vi "CRYPlot Polar Graph.vi"(7 "pGraph VI In":refnum<vi>, 8 "sOption":string, 9 "GraphSet":bool, 10 "Flattened Polar Property":string="Polar Property", 11 "Selected Rows In":i32[](array[numeric])) -> (0 "ItemSyms":i32[](array[numeric]), 1 "Freq Color":u32[](array[numeric]), 2 "Freq Name":string[](array[string]), 3 "Selected Row Out":i32[](array[numeric]))   [LabVIEW 2013]
uses:
  CRYWindow/DataView/Control/CRYPolar Property.ctl
  Global/CRYCurve Library Global.vi
panel:
  in  "Polar Property":T1={"polar attributes"={"maximum"=2.0, "minimum"=0.0, "clip to min"=FALSE, "log"=FALSE, "grid color"=3381657, "plot color"=16711680, "fmt and prec"={"format"=enum."Decimal", "precision"=2}, "visible section"=4}, "Auto/Manual"=0, "Zero Adjust (deg)"=0, "Angle Increment (deg)"=0, "Mirror"=FALSE, "Auto Increment"=FALSE, "Total Rotatin (deg)"=0, "Discrete/Rannge"=0, "Show Name"=FALSE, "CurValues"=[], "CurIndex"=0, "CurColors"=[], "CurColors_Range"=[], "CurValues_Range"=[], "Pen"={"Width"=1, "Style"=enum."Solid"}, "BackgroundColor"=0} {"polar attributes"."minimum" format="%0.2f"; "polar attributes"."maximum" format="%0.2f"}
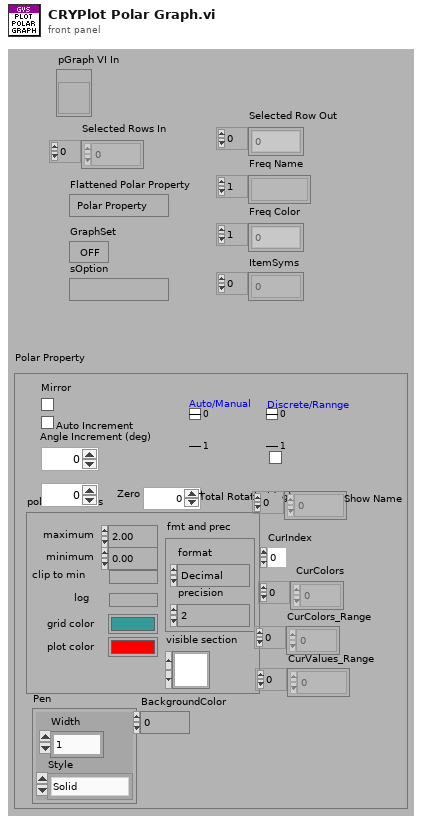
[diagram p1: front panel]
types:
  T1 = typedef "CRYPolar Property.ctl" = cluster{"polar attributes":cluster{"maximum":dbl, "minimum":dbl, "clip to min":bool, "log":bool, "grid color":u32, "plot color":u32, "fmt and prec":cluster{"format":enum8{"Decimal", "Scientific", "Engineering", "Binary", "Octal", "Hex"}, "precision":u8}, "visible section":u16}, "Auto/Manual":u16, "Zero Adjust (deg)":i32, "Angle Increment (deg)":i32, "Mirror":bool, "Auto Increment":bool, "Total Rotatin (deg)":i32, "Discrete/Rannge":u16, "Show Name":bool, "CurValues":dbl[], "CurIndex":u16, "CurColors":u32[], "CurColors_Range":u32[], "CurValues_Range":dbl[], "Pen":cluster{"Width":u16, "Style":enum32{"Solid", "Dash", "Dot", "DashDot", "DashDotDot"}}, "BackgroundColor":u32}
  T2 = cluster{"left":i16, "top":i16, "right":i16, "bottom":i16}
  T3 = typedef "CRYData Cluster.ctl" = cluster{"Name":string, "Curve":cluster{"x":dbl, "y":dbl, "z":dbl}[], "X data":u16, "Y data":u16, "Z data":u16, "X axis":u16, "Y axis":u16, "Z axis":u16, "X unit":string, "Y unit":string, "Z unit":string, "X dB ref":dbl, "Y dB ref":dbl, "Z dB ref":dbl, "single val":bool, "protected":bool, "display X":bool, "display Y":bool, "display Z":bool, "Test Info":string, "Step No.":i32, "Plot Settings":cluster{"Color":u32, "Interpolation":u8, "Point Style":u8, "Line Style":u8, "Point Color":u32, "Line Width":u8, "Bar Plot Style":u8, "Fill To":i16}, "AutoProtect":bool}
  T4 = cluster{"maximum":dbl, "minimum":dbl, "clip to min":bool, "log":bool, "grid color":u32, "plot color":u32, "fmt and prec":cluster{"format":enum8{"Decimal", "Scientific", "Engineering", "Binary", "Octal", "Hex"}, "precision":u8}, "visible section":u16}
  T5 = cluster{"Width":u16, "Style":enum32{"Solid", "Dash", "Dot", "DashDot", "DashDotDot"}}
  T6 = typedef "LVBoundsTypeDef.ctl" = cluster{"Width":u32, "Height":u32}
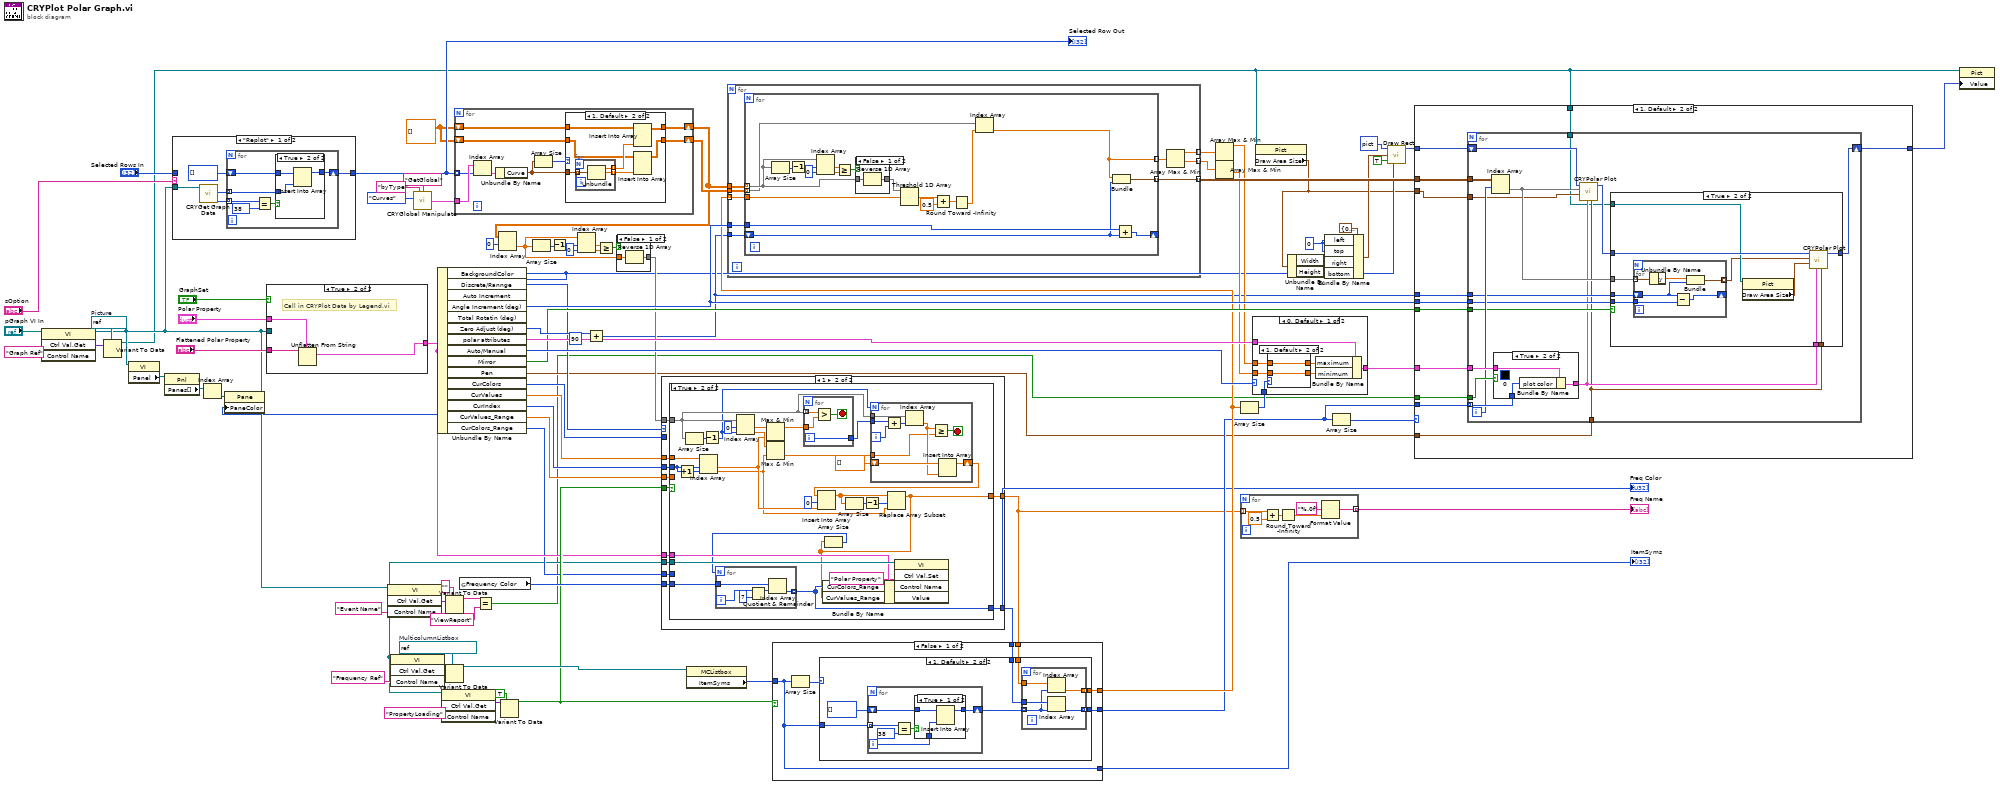
[diagram p0: block diagram]
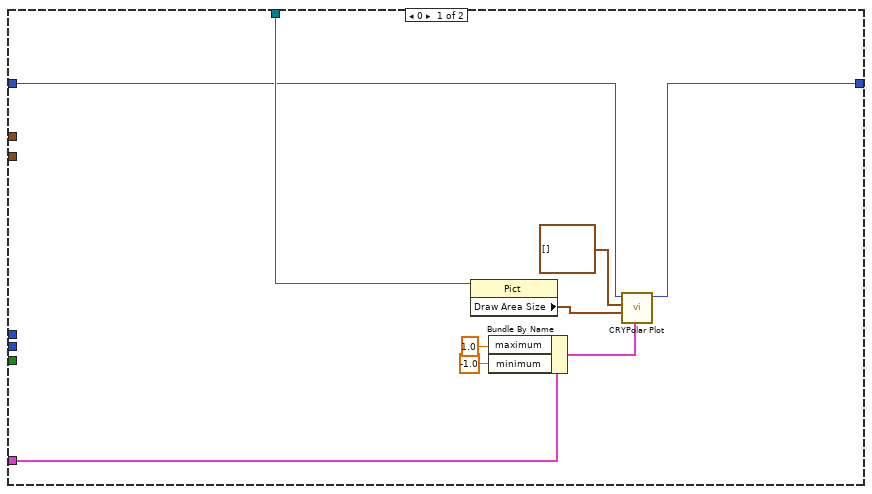
[diagram p6: hidden frame]
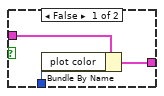
[diagram p8: hidden frame]
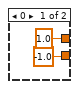
[diagram p11: hidden frame]
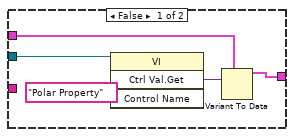
[diagram p17: hidden frame]
diagram:
  w13 = i16 0 ("left")
  w25 = refnum<vi> refnum  # Picture
  w32 = dbl[][] []
  w70 = refnum<vi> refnum  # MulticolumnListbox
  n1 = invoke class="VI" method="Ctrl Val.Get"(reference="pGraph VI In", "Control Name"="Graph Ref") -> (reference out=w21:refnum<vi>, "Get Control Value Variant"=w24:variant)  [unwired: 2 in, 2 out]
  n2 = Variant To Data(type=w25, Variant=w24) -> (data=w9:refnum<vi>)  [unwired: 1 in, 1 out]
  n3 = property class="VI"(reference=w21) -> ("Panel"=w19:refnum<vi>)  [unwired: 1 in, 2 out]
  n4 = property class="Pnl"(reference=w19) -> ("Panes[]"=w18:refnum<vi>[])  [unwired: 1 in, 2 out]
  n5 = case shown="\"Replot\"" "sOption" {
    tunnel: w21 -> [w89 _]
    tunnel: [w88 w103] -> w67
    tunnel: "Selected Rows In" -> [_ w103]
    frame "Replot" {
      n6 = call "CRYGet Graph Data.vi"("pGraph VI"=w89) -> ("Item Symbols"=w91:i32[], "Rows"=w92:i32[])  [unwired: 2 in, 7 out]
      n7 = for {
        tunnel: w91 -> [w97] mode=indexing
        tunnel: w92 -> [w95] mode=indexing
        shift-right: [w93] -> w88
        shift-left: i32[] [] ("Rows") -> [w94]
        n8 = Equal?(x=w97, y=38) -> (x = y?=w96:bool)
        n9 = case shown="True" w96 {
          tunnel: w95 -> [_ w100]
          tunnel: w94 -> [w99 w102]
          tunnel: [w99 w101] -> w93
          frame False {
          }
          frame True {
            n10 = Insert Into Array(array=w102, new element=w100) -> (w101:i32[])  [unwired: 1 in]
          }
        }
      }
    }
    frame "SameDrop", Default {
    }
  }
  "Selected Row Out" <- w67
  n11 = Index Array(array=w18) -> (element=w17:refnum<vi>)  [unwired: 1 in]
  n12 = case shown="True" "GraphSet" {
    tunnel: [w108 w109] -> w59
    tunnel: "Polar Property" -> [w107 w110]
    tunnel: w21 -> [w106 _]
    tunnel: "Flattened Polar Property" -> [_ w111]
    frame False {
      n13 = invoke class="VI" method="Ctrl Val.Get"(reference=w106, "Control Name"="Polar Property") -> ("Get Control Value Variant"=w104:variant)  [unwired: 2 in, 3 out]
      n14 = Variant To Data(type=w107, Variant=w104) -> (data=w108:T1)  [unwired: 1 in, 1 out]
    }
    frame True {
      # "Call in CRYPlot Data by Legend.vi"
      n15 = Unflatten From String(type=w110, binary string=w111) -> (value=w109:T1)  [unwired: 3 in, 2 out]
    }
  }
  n16 = invoke class="VI" method="Ctrl Val.Get"(reference=w21, "Control Name"="Event Name") -> ("Get Control Value Variant"=w83:variant)  [unwired: 2 in, 3 out]
  n17 = invoke class="VI" method="Ctrl Val.Get"(reference=w21, "Control Name"="Frequency Ref") -> ("Get Control Value Variant"=w71:variant)  [unwired: 2 in, 3 out]
  n18 = call "CRYGlobal Manipulate.vi"("Type"=enum16{"Curves", "Values", "Results", "WFM"}."Curves", "sOption"="byType", "sAction"="GetGlobal") -> ("Curves Out"=w1:T3[])  [unwired: 6 in, 6 out]
  n19 = Unbundle By Name(w59) -> ("BackgroundColor"=w7:u32, "Discrete/Rannge"=w73:u16, "Angle Increment (deg)"=w79:i32, "Zero Adjust (deg)"=w78:i32, "polar attributes"=w77:T4, "Auto/Manual"=w76:u16, "Mirror"=w75:bool, "Pen"=w28:T5, "CurColors"=w29:u32[], "CurValues"=w74:dbl[], "CurIndex"=w61:u16, "CurValues_Range"=w60:dbl[], "CurColors_Range"=w58:u32[])  [unwired: 2 out]
  n20 = property class="Pane"(reference=w17, "PaneColor"=w7) -> ()  [unwired: 1 in, 2 out]
  n21 = invoke class="VI" method="Ctrl Val.Get"(reference=w21, "Control Name"="PropertyLoading") -> ("Get Control Value Variant"=w64:variant)  [unwired: 2 in, 3 out]
  n22 = Variant To Data(type=w70, Variant=w71) -> (data=w69:refnum<vi>)  [unwired: 1 in, 1 out]
  n23 = Variant To Data(type="" ("Control Name"), Variant=w83) -> (data=w81:string)  [unwired: 1 in, 1 out]
  n24 = for {
    tunnel: w1 -> [w120]
    tunnel: w67 -> [w119] mode=indexing
    shift-right: [w113] -> w30
    shift-left: w32 -> [w115]
    shift-right: [w112] -> w31
    shift-left: w32 -> [w114]
    n25 = Index Array(array=w120, index=w119) -> (element=w118:T3)
    n26 = Unbundle By Name(w118) -> ("Curve"=w117:cluster{"x":dbl, "y":dbl, "z":dbl}[])
    n27 = Array Size(array=w117) -> (size(s)=w116:i32)
    n28 = case shown="1, Default" w116 {
      tunnel: w117 -> [_ w129]
      tunnel: w115 -> [w122 w128]
      tunnel: w114 -> [w121 w126]
      tunnel: [w122 w124] -> w113
      tunnel: [w121 w123] -> w112
      frame 0 {
      }
      frame 1, Default {
        n29 = for {
          tunnel: w129 -> [w132] mode=indexing
          tunnel: [w131] -> w125 mode=indexing
          tunnel: [w130] -> w127 mode=indexing
          n30 = Unbundle(w132) -> ("x"=w130:dbl, "y"=w131:dbl)  [unwired: 1 out]
        }
        n31 = Insert Into Array(array=w128, new element=w127) -> (w124:dbl[][])  [unwired: 2 in]
        n32 = Insert Into Array(array=w126, new element=w125) -> (w123:dbl[][])  [unwired: 2 in]
      }
    }
  }
  n33 = global read "CRYCurve Library Global.vi" "Frequency Color"() -> (w68:u32[])
  n34 = Equal?(x=w81, y="ViewReport" ("regular expression")) -> (x = y?=w20:bool)
  n35 = Index Array(array=w30, index (row)=0) -> (element=w34:dbl[])  [unwired: 1 in]
  n36 = Variant To Data(type=TRUE, Variant=w64) -> (data=w62:bool)  [unwired: 1 in, 1 out]
  n37 = Array Size(array=w34) -> (size(s)=w35:i32)
  n38 = Decrement(x=w35) -> (x-1=w36:i32)
  n39 = Index Array(array=w34, index #1=w36, index #2=0 ("index")) -> (element #1=w39:dbl, element #2=w38:dbl)
  n40 = Add(x=w78, y=90) -> (x+y=w27:i32)
  n41 = Greater Or Equal?(x=w39, y=w38) -> (x >= y?=w40:bool)
  n42 = case shown="False" w40 {
    tunnel: w34 -> [w134 w135]
    tunnel: [w133 w135] -> w33
    frame False {
      n43 = Reverse 1D Array(array=w134) -> (reversed array=w133:dbl[])
    }
    frame True {
    }
  }
  n44 = case shown="1" w73 {
    tunnel: w74 -> [w137 w147]
    tunnel: w29 -> [w136 _]
    tunnel: w68 -> [_ w146]
    tunnel: [w137 w142] -> w44
    tunnel: w61 -> [_ w148]
    tunnel: [w136 w145] -> w43
    tunnel: w62 -> [_ w139]
    tunnel: w58 -> [_ w140]
    tunnel: w21 -> [_ w144]
    tunnel: w59 -> [_ w143]
    tunnel: w60 -> [_ w141]
    tunnel: w33 -> [_ w138]
    frame 0, Default {
    }
    frame 1 {
      n45 = case shown="True" w139 {
        tunnel: w148 -> [_ w171]
        tunnel: w147 -> [_ w178]
        tunnel: w146 -> [_ w177]
        tunnel: [w149 w176] -> w145
        tunnel: w144 -> [_ w175]
        tunnel: w143 -> [_ w174]
        tunnel: [w150 w152] -> w142
        tunnel: w141 -> [w150 _]
        tunnel: w140 -> [w149 _]
        tunnel: w138 -> [_ w162]
        frame False {
        }
        frame True {
          n46 = Increment(x=w171) -> (x+1=w170:u16)
          n47 = Array Size(array=w162) -> (size(s)=w167:i32)
          n48 = Index Array(array=w178, index #1=w171, index #2=w170) -> (element #1=w156:dbl, element #2=w154:dbl)
          n49 = Decrement(x=w167) -> (x-1=w160:i32)
          n50 = Index Array(array=w162, index #1=0 ("index"), index #2=w160) -> (element #1=w168:dbl, element #2=w166:dbl)
          n51 = Max & Min(x=w168, y=w156) -> (max(x,y)=w163:dbl)  [unwired: 1 out]
          n52 = Max & Min(x=w166, y=w154) -> (min(x,y)=w164:dbl)  [unwired: 1 out]
          n53 = for {
            tunnel: w163 -> [w190]
            tunnel: w162 -> [w191] mode=indexing
            tunnel: [w188] -> w165
            i -> [w188]
            stop <- w189 stop-if-true
            n54 = Greater?(x=w191, y=w190) -> (0:w189:bool)
          }
          n55 = for {
            N: w160 -> [_]
            tunnel: w162 -> [w187]
            tunnel: w165 -> [w186]
            tunnel: w164 -> [w179]
            shift-right: [w182] -> w157
            shift-left: dbl[] [] -> [w183]
            i -> [w181]
            stop <- w184 stop-if-true
            n56 = Add(x=w186, y=w181) -> (x+y=w185:i32)
            n57 = Index Array(array=w187, index=w185) -> (element=w180:dbl)
            n58 = Greater Or Equal?(x=w180, y=w179) -> (x >= y?=w184:bool)
            n59 = Insert Into Array(array=w183, new element=w180) -> (w182:dbl[])  [unwired: 1 in]
          }
          n60 = Insert Into Array(array=w157, index=0, new element=w156) -> (w151:dbl[])
          n61 = Array Size(array=w151) -> (size(s)=w155:i32)
          n62 = Decrement(x=w155) -> (x-1=w153:i32)
          n63 = Replace Array Subset(array=w151, new element=w154, index=w153) -> (w152:dbl[])
          n64 = Array Size(array=w152) -> (size(s)=w161:i32)
          n65 = for {
            N: w161 -> [_]
            tunnel: w177 -> [w194]
            tunnel: [w193] -> w176 mode=indexing
            i -> [w192]
            n66 = Quotient & Remainder(x=w192, y=7) -> (x-y*floor(x/y)=w196:i32)  [unwired: 1 out]
            n67 = Index Array(array=w194, index=w196) -> (element=w193:u32)
          }
          n68 = Bundle By Name(cluster=w174, "CurColors_Range"=w176, "CurValues_Range"=w152) -> (w172:T1)
          n69 = invoke class="VI" method="Ctrl Val.Set"(reference=w175, "Control Name"="Polar Property", "Value"=w172) -> ()  [unwired: 2 in, 5 out]
        }
      }
    }
  }
  "Freq Color" <- w43
  n70 = property on="Property Node" class="MCListbox"(reference=w69) -> ("ItemSyms"=w42:i32[])  [unwired: 1 in, 2 out]
  n71 = case shown="False" w62 {
    tunnel: [w202 w229] -> w48
    tunnel: w44 -> [w200 w229]
    tunnel: [w199 w228] -> w46
    tunnel: w43 -> [w198 w228]
    tunnel: [w197 w227] -> w45
    tunnel: w42 -> [w197 w227]
    frame False {
      n72 = Array Size(array=w197) -> (size(s)=w201:i32)
      n73 = case shown="1, Default" w201 {
        tunnel: w200 -> [w204 w211]
        tunnel: [w204 w210] -> w202
        tunnel: w198 -> [w203 w209]
        tunnel: [w203 w208] -> w199
        tunnel: w197 -> [_ w205]
        frame 0 {
        }
        frame 1, Default {
          n74 = for {
            tunnel: w205 -> [w221] mode=indexing
            shift-right: [w218] -> w206
            shift-left: i32[] [] ("Rows") -> [w219]
            i -> [w217]
            n75 = Equal?(x=w221, y=38) -> (x = y?=w220:bool)
            n76 = case shown="True" w220 {
              tunnel: w219 -> [w225 w226]
              tunnel: [w224 w226] -> w218
              tunnel: w217 -> [w223 _]
              frame True {
                n77 = Insert Into Array(array=w225, new element=w223) -> (w224:i32[])  [unwired: 1 in]
              }
              frame False {
              }
            }
          }
          n78 = for {
            tunnel: w206 -> [w212] mode=indexing
            tunnel: w211 -> [w216]
            tunnel: [w215] -> w210 mode=indexing
            tunnel: w209 -> [w214]
            tunnel: [w213] -> w208 mode=indexing
            n79 = Index Array(array=w216, index=w212) -> (element=w215:dbl)
            n80 = Index Array(array=w214, index=w212) -> (element=w213:u32)
          }
        }
      }
    }
    frame True {
      # "Property dialog has been currently loaded"
    }
  }
  "ItemSyms" <- w45
  n81 = for {
    tunnel: w27 -> [w238]
    tunnel: w79 -> [w237]
    tunnel: w48 -> [w236] mode=indexing
    tunnel: w31 -> [w235]
    tunnel: [w234] -> w55 mode=indexing
    tunnel: [w232] -> w54 mode=indexing
    tunnel: [w231] -> w53 mode=indexing
    tunnel: w30 -> [w230]
    n82 = for {
      tunnel: w235 -> [w240] mode=indexing
      tunnel: w236 -> [w243]
      tunnel: w237 -> [w247]
      shift-right: [w246] -> _
      shift-left: w238 -> [w245]
      tunnel: [w244] -> w234 mode=indexing
      tunnel: [w239] -> w233 mode=indexing
      tunnel: w230 -> [w241] mode=indexing
      n83 = Array Size(array=w241) -> (size(s)=w257:i32)
      n84 = Decrement(x=w257) -> (x-1=w256:i32)
      n85 = Index Array(array=w241, index #1=w256, index #2=0 ("index")) -> (element #1=w253:dbl, element #2=w254:dbl)
      n86 = Greater Or Equal?(x=w253, y=w254) -> (x >= y?=w249:bool)
      n87 = case shown="False" w249 {
        tunnel: w241 -> [w259 w260]
        tunnel: [w258 w260] -> w242
        frame False {
          n88 = Reverse 1D Array(array=w259) -> (reversed array=w258:dbl[])
        }
        frame True {
        }
      }
      n89 = Threshold 1D Array(2:w243, 3:w242) -> (0:w252:dbl)  [unwired: 1 in]
      n90 = Add(x=w252, y=0.5) -> (x+y=w250:dbl)
      n91 = Round Toward -Infinity(1:w250) -> (0:w248:dbl)
      n92 = Index Array(array=w240, index=w248) -> (element=w239:dbl)
      n93 = Bundle("y"=w239, w245) -> (w244:cluster{"y":dbl, i32})  [unwired: 1 out]
      n94 = Add(x=w247, y=w245) -> (x+y=w246:i32)
    }
    n95 = Array Max & Min(array=w233) -> (max value=w232:dbl, min value=w231:dbl)  [unwired: 2 out]
  }
  n96 = Array Max & Min(array=w54) -> (max value=w51:dbl)  [unwired: 3 out]
  n97 = Array Max & Min(array=w53) -> (min value=w50:dbl)  [unwired: 3 out]
  n98 = Array Size(array=w48) -> (size(s)=w49:i32)
  n99 = for {
    tunnel: w44 -> [w261] mode=indexing
    tunnel: [w265] -> w56 mode=indexing
    n100 = Add(x=w261, y=0.5) -> (x+y=w263:dbl)
    n101 = Round Toward -Infinity(1:w263) -> (0:w262:dbl)
    n102 = Format Value(format string="%.0f", value (0)=w262) -> (output string=w265:string)  [unwired: 1 in]
  }
  "Freq Name" <- w56
  n103 = case shown="0, Default" w76 {
    tunnel: [w273 w278] -> w52
    tunnel: w51 -> [w269 _]
    tunnel: w50 -> [w267 _]
    tunnel: w77 -> [w272 w278]
    tunnel: w49 -> [w271 _]
    frame 0, Default {
      n104 = case shown="1, Default" w271 {
        tunnel: [1.0 w277] -> w270
        tunnel: w269 -> [_ w277]
        tunnel: [-1.0 w276] -> w268
        tunnel: w267 -> [_ w276]
        frame 0 {
        }
        frame 1, Default {
        }
      }
      n105 = Bundle By Name(cluster=w272, "maximum"=w270, "minimum"=w268) -> (w273:T4)
    }
    frame 1 {
    }
  }
  n106 = property class="Pict"(reference=w9) -> ("Draw Area Size"=w5:T6)  [unwired: 1 in, 2 out]
  n107 = Unbundle By Name(w5) -> ("Width"=w14:u32, "Height"=w15:u32)
  n108 = Bundle By Name(cluster=T2 {"left"=0, "top"=0, "right"=0, "bottom"=0} ("rect"), "left"=w13, "top"=w13, "right"=w14, "bottom"=w15) -> (w8:T2)
  n109 = Array Size(array=w46) -> (size(s)=w47:i32)
  n110 = call <vilib>:"Draw Rect.vi"("picture"=picture data[5B] ("Value"), "rect"=w8, "fill?(F)"=TRUE, "color(black)"=w7) -> ("new picture"=w6:picture)  [unwired: 5 in]
  n111 = case shown="1, Default" w47 {
    tunnel: [w281 w299] -> w57
    tunnel: w20 -> [_ w298]
    tunnel: w9 -> [w282 w290]
    tunnel: w27 -> [_ w297]
    tunnel: w79 -> [_ w296]
    tunnel: w75 -> [_ w292]
    tunnel: w55 -> [_ w295]
    tunnel: w52 -> [w280 w294]
    tunnel: w46 -> [_ w293]
    tunnel: w28 -> [_ w291]
    tunnel: w6 -> [w279 w288]
    tunnel: w5 -> [_ w289]
    frame 0 {
      n112 = property class="Pict"(reference=w282) -> ("Draw Area Size"=w287:T6)  [unwired: 1 in, 2 out]
      n113 = Bundle By Name(cluster=w280, "maximum"=1.0, "minimum"=-1.0) -> (w285:T4)
      n114 = call "CRYPolar Plot.vi"("polar attributes"=w285, "dimensions (w,h)"=w287, "data array [mag, phase (deg)]"=cluster{"magnitude":dbl, "phase":dbl}[] [], "picture"=w279) -> ("new picture"=w281:picture)  [unwired: 1 in, 6 out]
    }
    frame 1, Default {
      n115 = for {
        tunnel: w298 -> [w315]
        tunnel: w290 -> [w300]
        tunnel: w294 -> [w314]
        tunnel: w297 -> [w307]
        tunnel: w296 -> [w306]
        tunnel: w295 -> [w311]
        shift-right: [w304] -> w299
        shift-left: w288 -> [w313]
        tunnel: w293 -> [w312] mode=indexing
        tunnel: w292 -> [w308]
        tunnel: w291 -> [w302]
        tunnel: w289 -> [w301]
        i -> [w310]
        n116 = Index Array(array=w311, index (row)=w310) -> (element=w309:cluster{"y":dbl, i32}[])  [unwired: 1 in]
        n117 = case shown="True" w315 {
          tunnel: w314 -> [w335 w338]
          tunnel: [w334 w337] -> w303
          tunnel: w312 -> [w333 w336]
          frame False {
            n118 = Bundle By Name(cluster=w335, "plot color"=w333) -> (w334:T4)
          }
          frame True {
            (unwired) u32 0
            n119 = Bundle By Name(cluster=w338, "plot color"=w336) -> (w337:T4)
          }
        }
        n120 = call "CRYPolar Plot.vi"("Pen"=w302, "polar attributes"=w303, "dimensions (w,h)"=w301, "data array [mag, phase (deg)]"=w309, "picture"=w313) -> ("new picture"=w305:picture)  [unwired: 6 out]
        n121 = case shown="True" w308 {
          tunnel: w307 -> [_ w326]
          tunnel: w306 -> [_ w325]
          tunnel: w309 -> [_ w324]
          tunnel: w305 -> [w316 w323]
          tunnel: [w316 w322] -> w304
          tunnel: w300 -> [_ w321]
          tunnel: w303 -> [_ w318]
          tunnel: w302 -> [_ w317]
          frame False {
          }
          frame True {
            n122 = for {
              tunnel: w324 -> [w332] mode=indexing
              tunnel: [w330] -> w319 mode=indexing
              shift-right: [w328] -> _
              shift-left: w326 -> [w327]
              tunnel: w325 -> [w329]
              n123 = Unbundle By Name(w332) -> ("y"=w331:dbl)
              n124 = Subtract(x=w327, y=w329) -> (x-y=w328:i32)
              n125 = Bundle("y"=w331, w327) -> (w330:cluster{"y":dbl, i32})  [unwired: 1 out]
            }
            n126 = property class="Pict"(reference=w321) -> ("Draw Area Size"=w320:T6)  [unwired: 1 in, 2 out]
            n127 = call "CRYPolar Plot.vi"("Pen"=w317, "polar attributes"=w318, "dimensions (w,h)"=w320, "data array [mag, phase (deg)]"=w319, "picture"=w323) -> ("new picture"=w322:picture)  [unwired: 6 out]
          }
        }
      }
    }
  }
  n128 = property class="Pict"(reference=w9, "Value"=w57) -> ()  [unwired: 1 in, 2 out]
